vi "Get Parent Index.vi"(8 "Error In":errorcluster, 11 "reference in":refnum<class "OD Sub-Entry.lvclass">) -> (0 "Error Out":errorcluster, 2 "Parent Index":u16 format="%.0x", 3 "reference out":refnum<class "OD Sub-Entry.lvclass">)   [LabVIEW 2019, in "Electronic Datasheet.lvlib" / "OD Sub-Entry.lvclass"]
uses:
  OD Sub-Entry.lvclass
  OD Sub-Entry.lvclass/OD Sub-Entry.ctl
  OD Entry/OD Entry.lvclass
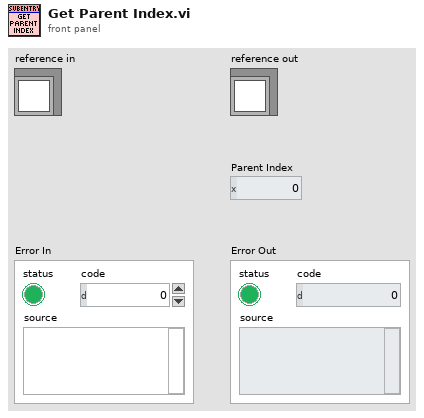
[diagram p1: front panel]
types:
  T1 = typedef "Electronic Datasheet.lvlib/OD Sub-Entry.lvclass/ObjectAttributes.ctl" = cluster{"Parent":refnum<class "OD Entry.lvclass">}
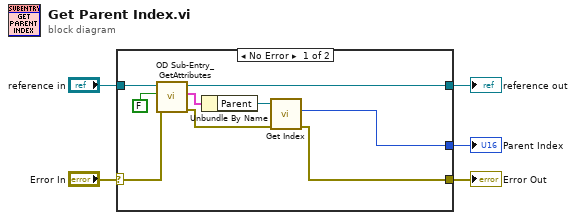
[diagram p0: block diagram]
diagram:
  n1 = case shown="No Error" "Error In" {
    selector: "Error In" -> [w14 w16]
    tunnel: [w7 w16] -> w4
    tunnel: [w12 w15] -> w2
    tunnel: "reference in" -> [w13 w15]
    tunnel: [w6 _] -> w1
    frame No Error {
      n2 = call "OD Sub-Entry_GetAttributes.vi"("Error In"=w14, "OnlyGetDvrReference(False)"=FALSE, "reference in"=w13) -> ("Error Out"=w8:errorcluster, "Data"=w10:T1, "reference out"=w12:refnum<class "OD Sub-Entry.lvclass">)  [unwired: 5 in, 1 out]
      n3 = Unbundle By Name(w10) -> ("Parent"=w9:refnum<class "OD Entry.lvclass">)
      n4 = call "Get Index.vi"("Error In"=w8, "reference in"=w9) -> ("Error Out"=w7:errorcluster, "Index"=w6:u16)  [unwired: 7 in, 1 out]
    }
    frame Error {
    }
  }
  "Error Out" <- w4
  "reference out" <- w2
  "Parent Index" <- w1
